vi "GxSingleCam.vi"() -> ()   [LabVIEW 2016]
uses:
  <vilib>/vision/Image Controls.llb/IMAQ Image.ctl
  GxLVLib/GxLVLib.lvlib
panel:
  in  "TriggerMode":string(combo)
  in  "Image Path":path
  in  "Image Src":T1
  out "IsColor":bool
  out "error out":errorcluster
  in  "DeviceHandle":u64
  out "IsExit":bool
  in  "ImageSaving":bool caption="保存图片"
  out "Acquisition Status":bool
  out "Open Status":bool
  in  "Exit":bool caption="安全退出"
  in  "TriggerSoftware":bool caption="发送软触发"
  in  "BalanceWhiteAuto":string(combo) caption="自动白平衡"
  in  "Gain":dbl caption="增益" format="%#_6f"
  in  "ExposureTime":dbl caption="曝光时间"
  in  "TriggerSource":string(combo) caption="触发源"
  in  "Acquisition Stop":bool caption="停止采集"
  in  "Acquisition Start":bool caption="开始采集"
  in  "Close Device":bool caption="关闭设备"
  in  "Open Device":bool caption="打开设备"
  out "Image":T1(plugin-control)
  # "TriggerMode"
  # "TriggerSource"
  # "TriggerSoftware"
  # "ExposureTime(us)"
  # "Gain(dB)"
  # "BalanceWhiteAuto"
  # "ImageSaving"
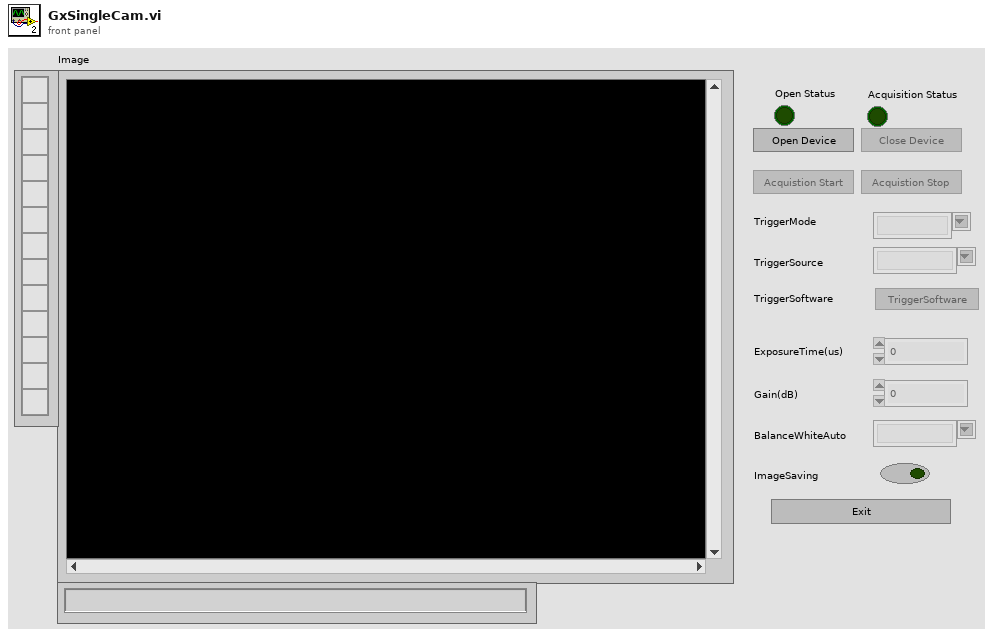
[diagram p1: front panel]
types:
  T1 = typedef "IMAQ Image.ctl" = refnum<image>
  T2 = typedef "Semaphore RefNum" = refnum<k1>
  T3 = cluster{"nFrameID":u64, "nTimestamp":u64, "nBufID":u64, "pImgBuf":u64, "nStatus":i32, "nWidth":i32, "nHeight":i32, "nPixelFormat":i32, "nImgSize":i32, "nOffsetX":i32, "nOffsetY":i32, "pUserParam":i32, cluster{"[0]":i32, "[1]":i32, "[2]":i32, "[3]":i32, "[4]":i32, "[5]":i32, "[6]":i32, "[7]":i32, "[8]":i32, "[9]":i32, "[10]":i32, "[11]":i32, "[12]":i32, "[13]":i32, "[14]":i32, "[15]":i32, "[16]":i32, "[17]":i32, "[18]":i32, "[19]":i32, "[20]":i32, "[21]":i32, "[22]":i32}}
  T4 = enum8{"Enabled", "Disabled", "Disabled and Grayed Out"}
  T5 = typedef "Image Type" = u32
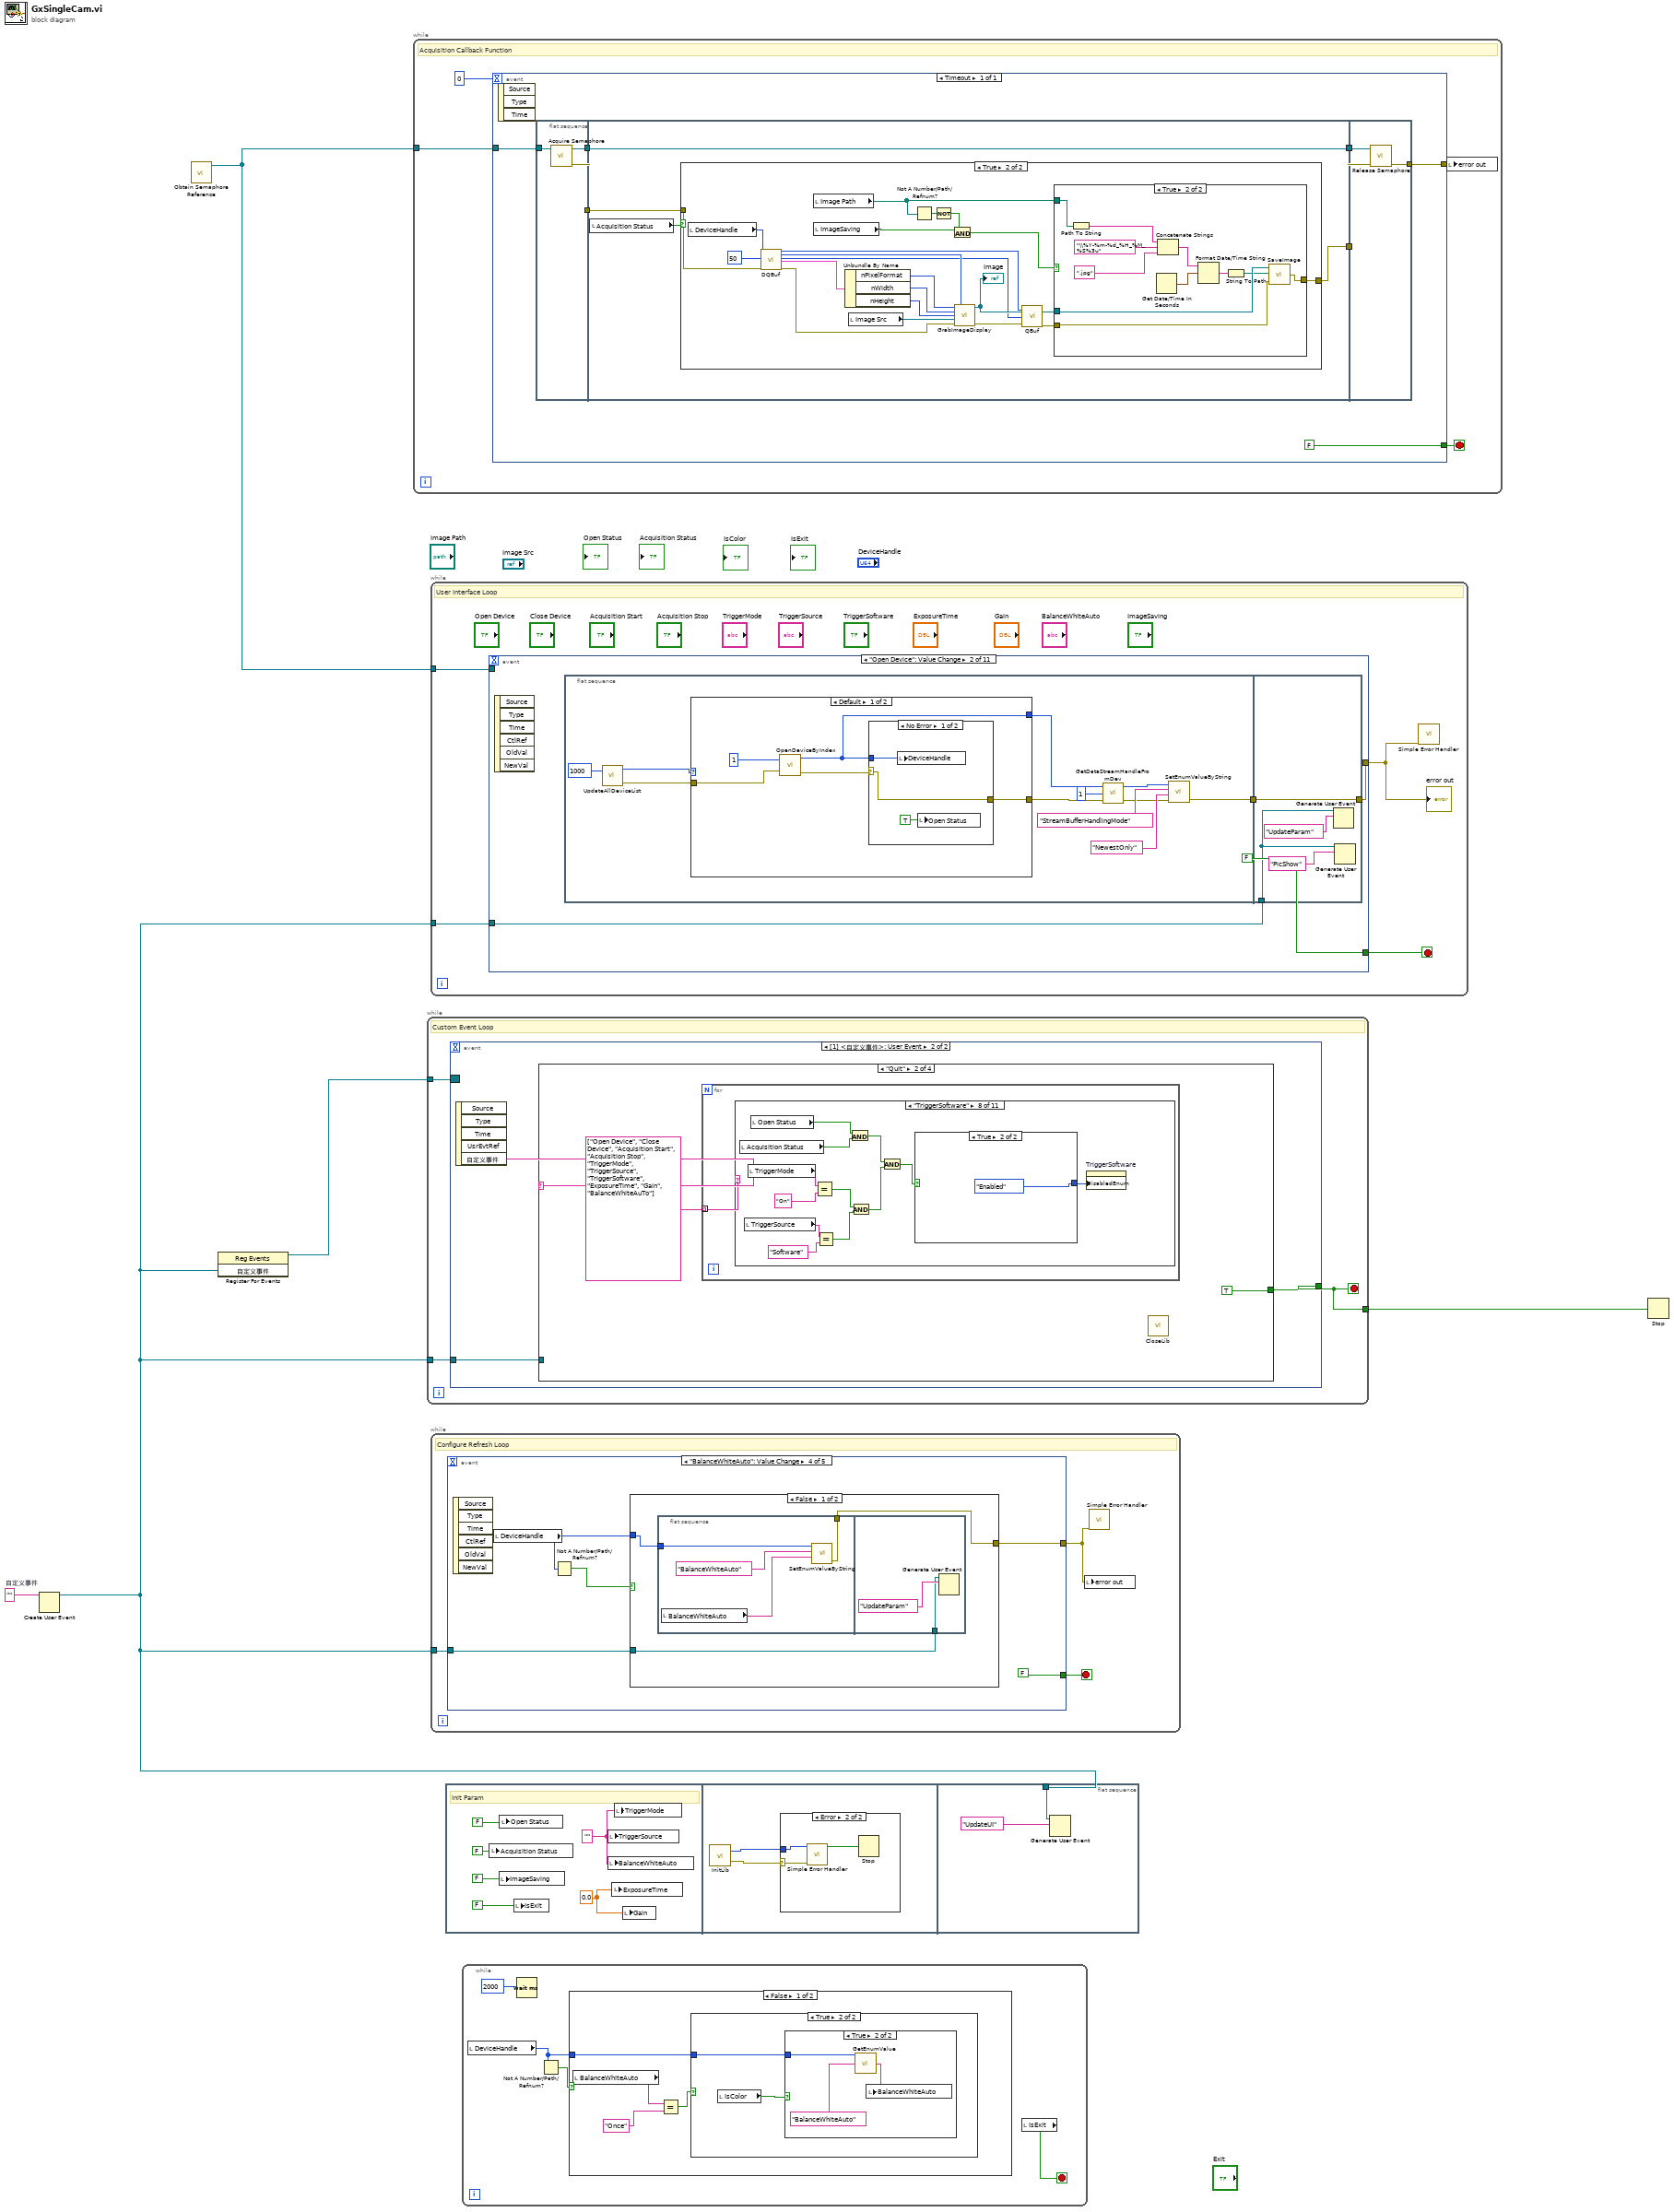
[diagram p0: block diagram]
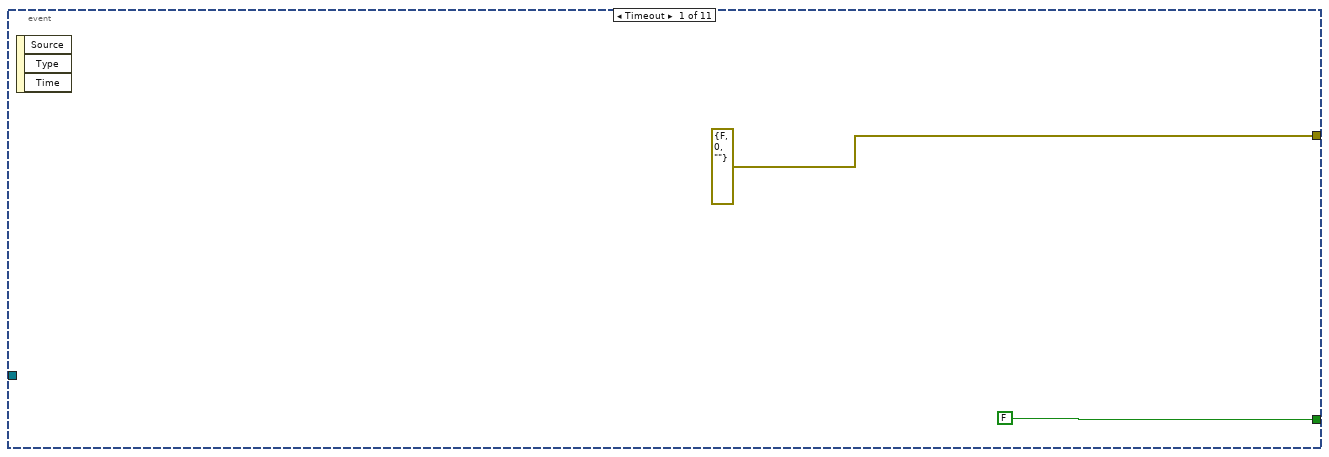
[diagram p4: hidden frame]
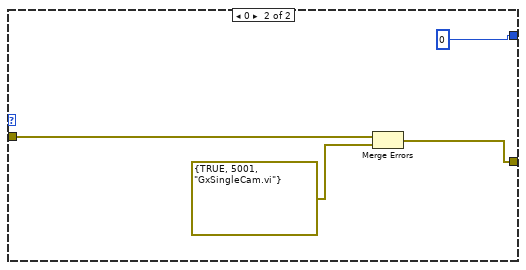
[diagram p6: hidden frame]
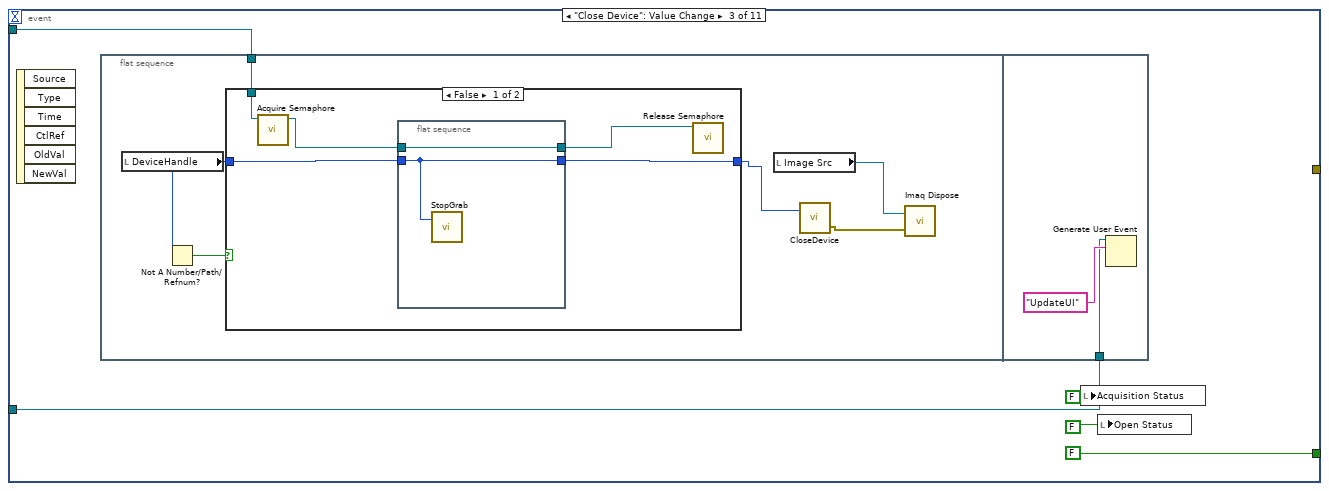
[diagram p7: hidden frame]
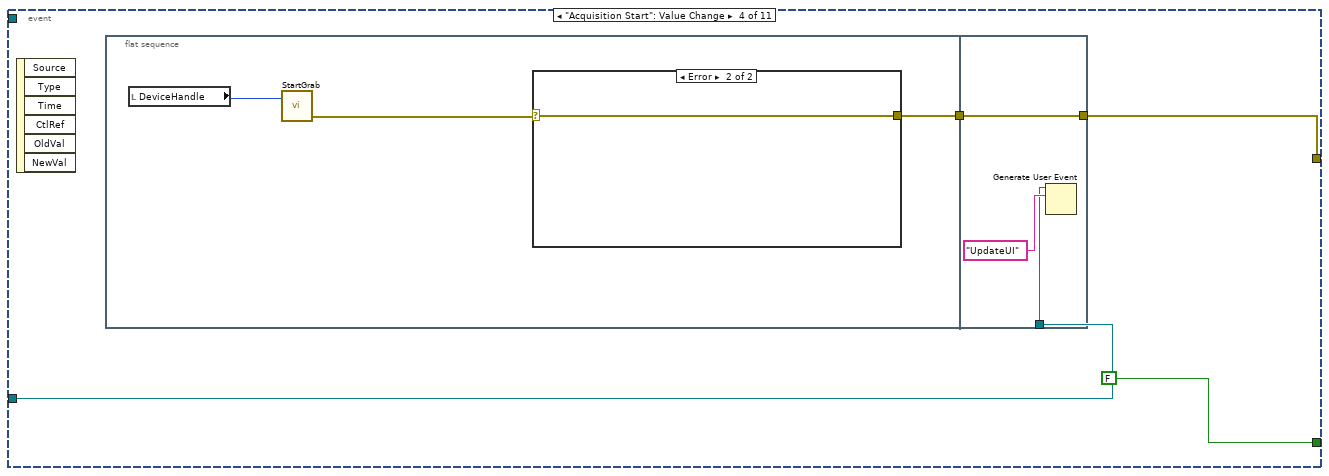
[diagram p9: hidden frame]
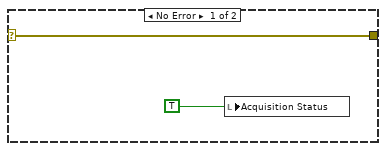
[diagram p10: hidden frame]
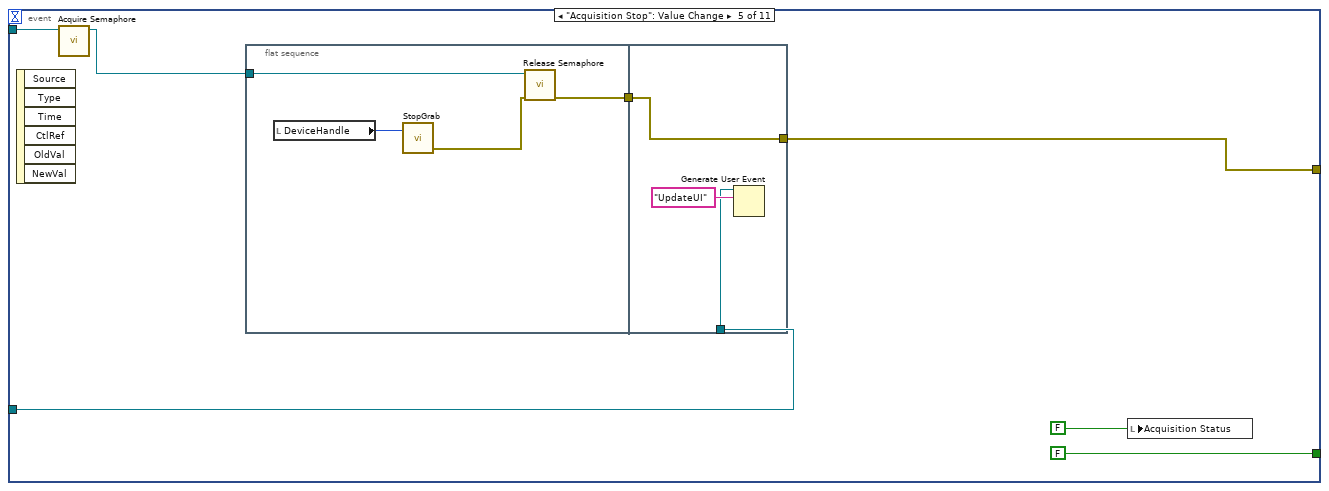
[diagram p11: hidden frame]
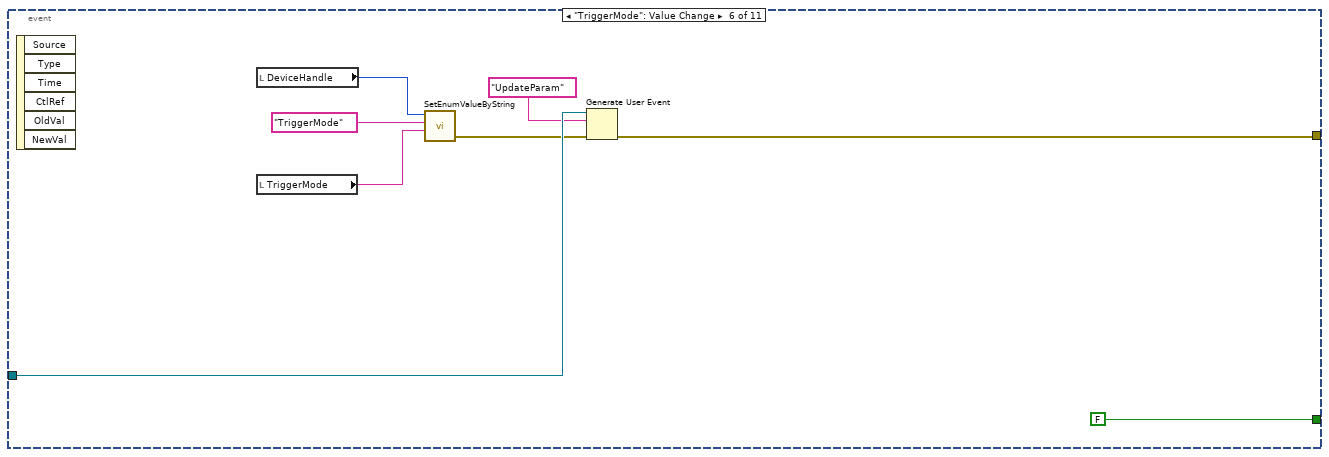
[diagram p12: hidden frame]
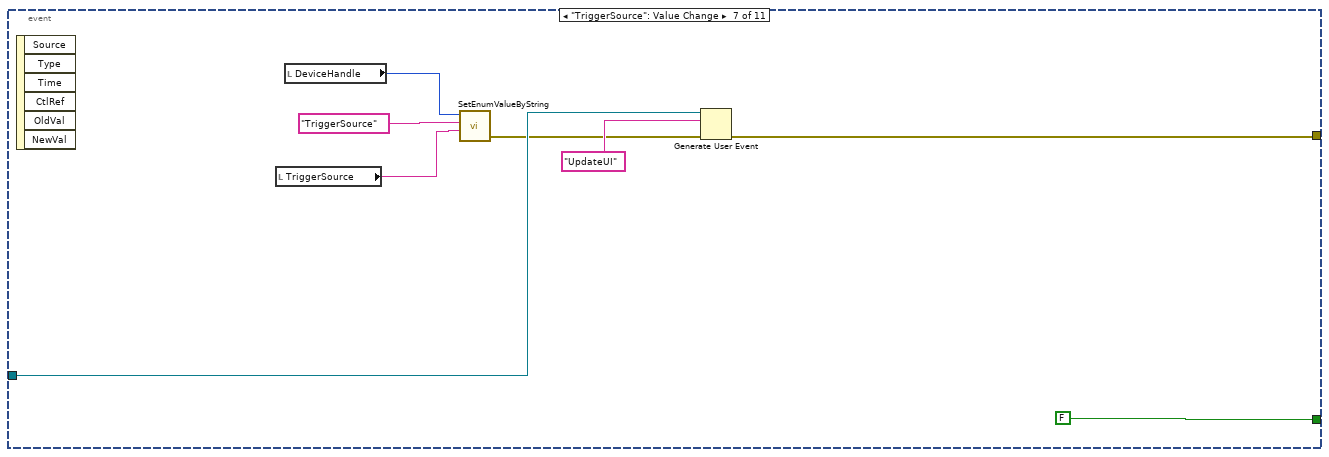
[diagram p13: hidden frame]
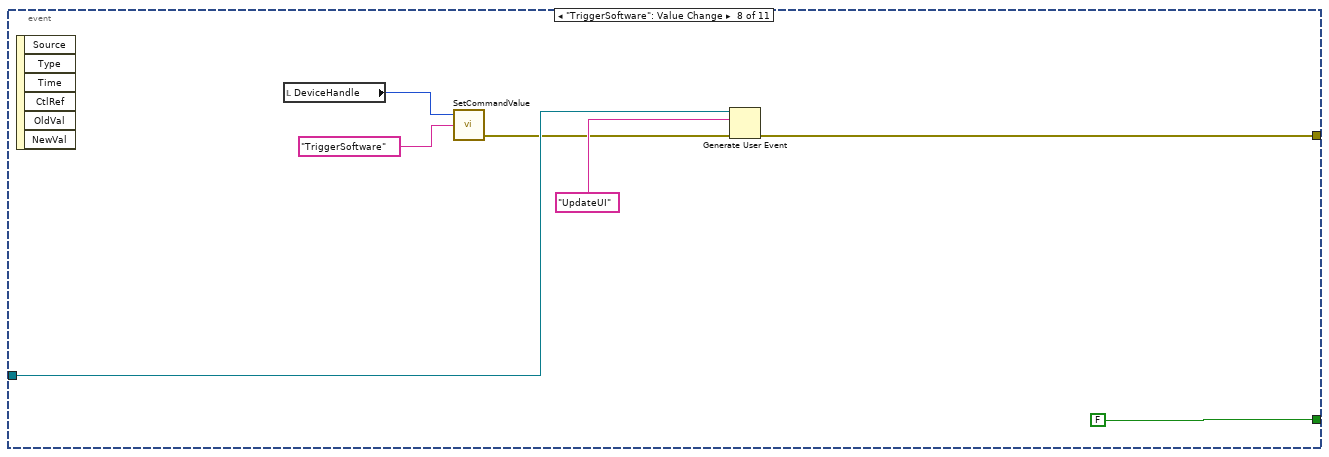
[diagram p14: hidden frame]
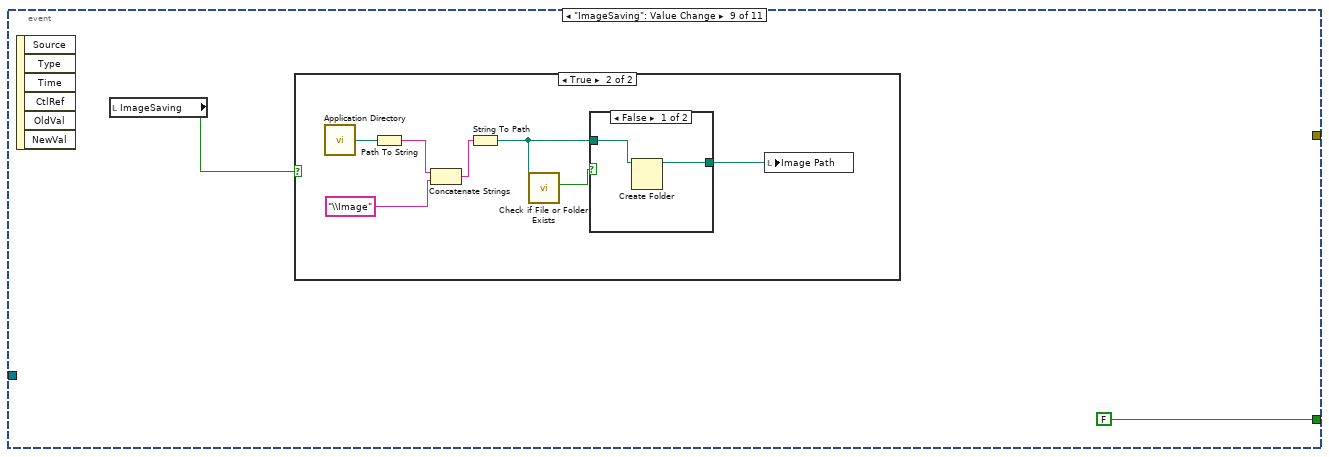
[diagram p15: hidden frame]
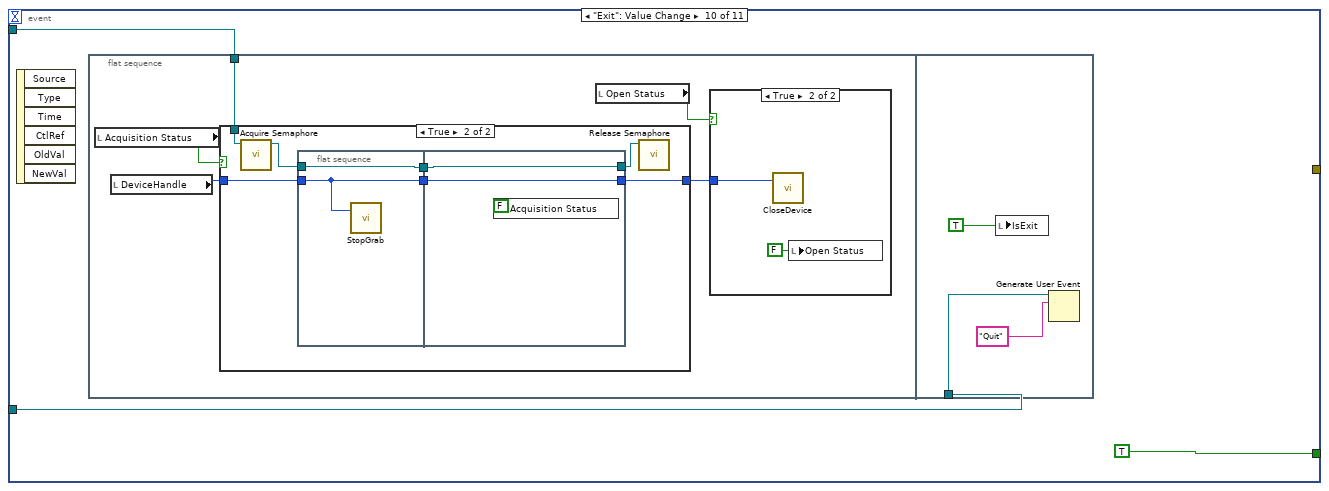
[diagram p18: hidden frame]
diagram:
  w5 = ""  # 自定义事件
  n1 = Create User Event(user event datatype=w5) -> (user event=w2:refnum<user-event>)  [unwired: 1 in, 1 out]
  n2 = call <vilib>:"Obtain Semaphore Reference.vi"() -> ("semaphore"=w1:T2)  [unwired: 5 in, 2 out]
  n3 = register-events(w2) -> (reference out=w4:refnum<event-registration>)  [unwired: 2 in, 1 out]
  n4 = while {
    tunnel: w1 -> [w6]
    stop <- w9 stop-if-true
    # "Acquisition Callback Function"
    n5 = event shown="[0] Timeout" {
      selector: _ -> [_]
      dyn-events: _ -> [_]
      timeout: 0 -> [_]
      tunnel: [FALSE] -> w9
      tunnel: [w15] -> w8
      tunnel: w6 -> [w14]
      event Timeout {
        n6 = event-data() -> ()  [unwired: 1 in, 3 out]
        n7 = flat-sequence {
          tunnel: w14 -> [w19]
          tunnel: [w18] -> w11
          tunnel: [w17] -> w10
          tunnel: [w23] -> w13
          tunnel: [w22] -> w12
          tunnel: w11 -> [w22]
          tunnel: w10 -> [w21]
          tunnel: [w58] -> w15
          tunnel: w13 -> [w59]
          tunnel: w12 -> [w60]
          frame #0 {
            n8 = call <vilib>:"Acquire Semaphore.vi"("semaphore"=w19) -> ("error out"=w17:errorcluster, "semaphore out"=w18:T2)  [unwired: 4 in, 1 out]
          }
          frame #1 {
            n9 = local read "Acquisition Status"() -> (w20:bool)
            n10 = case shown="True" w20 {
              tunnel: [w24 w40] -> w23
              tunnel: w21 -> [w24 w43]
              frame False {
              }
              frame True {
                n11 = local read "DeviceHandle"() -> (w45:u64)
                n12 = call "DQBuf.vi"("nInputHandle"=w45, "nTimeOut"=50, "error in (no error)"=w43) -> ("nOutputHandle"=w42:u64, "ImgBuf"=w32:u8[], "ppFrameBuffer"=w25:u64, "Dst"=w41:T3, "error out"=w28:errorcluster)  [unwired: 11 in, 1 out]
                n13 = local read "Image Path"() -> (w36:path)
                n14 = local read "ImageSaving"() -> (w35:bool)
                n15 = Unbundle By Name(w41) -> ("nPixelFormat"=w29:i32, "nWidth"=w31:i32, "nHeight"=w30:i32)
                n16 = local read "Image Src"() -> (w33:T1)
                n17 = Not A Number/Path/Refnum?(number/path/refnum=w36) -> (NaN/Path/Refnum?=w37:bool)
                n18 = Not(x=w37) -> (.not. x?=w38:bool)
                n19 = And(x=w35, y=w38) -> (x .and. y?=w34:bool)
                n20 = call "GrabImageDisplay.vi"("nPixelFormat"=w29, "pInputBuffer"=w32, "nWidth"=w31, "nHeight"=w30, "Image Src"=w33, "error in (no error)"=w28) -> ("Image out"=w27:T1, "error out"=w26:errorcluster)  [unwired: 8 in]
                "Image" <- w27
                n21 = call "QBuf.vi"("error in (no error)"=w26, "pBufferHandle"=w25, "nInputHandle"=w42) -> ("error out"=w39:errorcluster)  [unwired: 2 out]
                n22 = case shown="True" w34 {
                  tunnel: w36 -> [_ w53]
                  tunnel: w27 -> [_ w52]
                  tunnel: w39 -> [w46 w50]
                  tunnel: [w46 w49] -> w40
                  frame False {
                  }
                  frame True {
                    n23 = Path To String(path=w53) -> (string=w54:string)
                    n24 = Get Date/Time In Seconds() -> (seconds since 1Jan1904=w56:timestamp)
                    n25 = Concatenate Strings(w54, "\\%Y-%m-%d_%H_%M_%S%3u", ".jpg") -> (w55:string)
                    n26 = Format Date/Time String(time format string (%c)=w55, seconds (now)=w56) -> (date/time string=w57:string)  [unwired: 1 in]
                    n27 = String To Path(string=w57) -> (path=w51:path)
                    n28 = call "SaveImage.vi"("error in (no error)"=w50, "Path"=w51, "Image Src"=w52) -> ("error out"=w49:errorcluster)
                  }
                }
              }
            }
          }
          frame #2 {
            n29 = call <vilib>:"Release Semaphore.vi"("error in (no error)"=w59, "semaphore"=w60) -> ("error out"=w58:errorcluster)  [unwired: 4 in, 1 out]
          }
        }
      }
    }
    n30 = local write "error out"(w8) -> ()
  }
  n31 = while {
    tunnel: w4 -> [w63]
    tunnel: w2 -> [w62]
    tunnel: [w61] -> w3
    stop <- w61 stop-if-true
    # "Custom Event Loop"
    n32 = event shown="[1] <自定义事件>: User Event" {
      selector: w63 -> [_ _]
      dyn-events: _ -> [_ _]
      timeout: _ -> [_ _]
      tunnel: [FALSE w65] -> w61
      tunnel: w62 -> [_ w66]
      event Timeout {
        n33 = event-data() -> ()  [unwired: 1 in, 3 out]
      }
      event User Event {
        n34 = event-data() -> ("自定义事件"=w67:string)  [unwired: 1 in, 4 out]
        n35 = case shown="\"Quit\"" w67 {
          tunnel: w66 -> [_ _ w196 _]
          tunnel: [FALSE TRUE FALSE FALSE] -> w65
          frame "UpdateUI", Default {
            n36 = for {
              tunnel: string[] ["OpenDevice", "CloseDevice", "Acquisition Start", "Acquisition Stop", "TriggerMode", "TriggerSource", "TriggerSoftware", "ExposureTime", "Gain", "BalanceWhiteAuto"] -> [w70] mode=indexing
              n37 = case shown="\"BalanceWhiteAuto\"" w70 {
                frame Default {
                }
                frame "OpenDevice" {
                  n38 = local read "Open Status"() -> (w72:bool)
                  n39 = case shown="True" w72 {
                    tunnel: [T4."Enabled" ("禁用") T4."Disabled and Grayed Out" ("禁用")] -> w71
                    frame False {
                    }
                    frame True {
                    }
                  }
                  n40 = property on="Open Device" class="Bool"("DisabledEnum"=w71) -> ()  [unwired: 2 in, 2 out]
                }
                frame "CloseDevice" {
                  n41 = local read "Open Status"() -> (w76:bool)
                  n42 = case shown="True" w76 {
                    tunnel: [T4."Disabled and Grayed Out" ("禁用") T4."Enabled" ("禁用")] -> w75
                    frame False {
                    }
                    frame True {
                    }
                  }
                  n43 = property on="Close Device" class="Bool"("DisabledEnum"=w75) -> ()  [unwired: 2 in, 2 out]
                }
                frame "Acquisition Start" {
                  n44 = local read "Acquisition Status"() -> (w83:bool)
                  n45 = local read "Open Status"() -> (w82:bool)
                  n46 = Not(x=w83) -> (.not. x?=w81:bool)
                  n47 = And(x=w82, y=w81) -> (x .and. y?=w80:bool)
                  n48 = case shown="False" w80 {
                    tunnel: [T4."Disabled and Grayed Out" ("禁用") T4."Enabled" ("禁用")] -> w79
                    frame False {
                    }
                    frame True {
                    }
                  }
                  n49 = property on="Acquisition Start" class="Bool"("DisabledEnum"=w79) -> ()  [unwired: 2 in, 2 out]
                }
                frame "Acquisition Stop" {
                  n50 = local read "Acquisition Status"() -> (w87:bool)
                  n51 = case shown="False" w87 {
                    tunnel: [T4."Disabled and Grayed Out" ("禁用") T4."Enabled" ("禁用")] -> w86
                    frame False {
                    }
                    frame True {
                    }
                  }
                  n52 = property on="Acquisition Stop" class="Bool"("DisabledEnum"=w86) -> ()  [unwired: 2 in, 2 out]
                }
                frame "TriggerMode" {
                  n53 = local read "Open Status"() -> (w91:bool)
                  n54 = case shown="True" w91 {
                    tunnel: [T4."Disabled and Grayed Out" ("禁用") T4."Enabled" ("禁用")] -> w90
                    frame False {
                    }
                    frame True {
                    }
                  }
                  n55 = property on="TriggerMode" class="CmbBox"("DisabledEnum"=w90) -> ()  [unwired: 2 in, 2 out]
                }
                frame "TriggerSource" {
                  n56 = local read "TriggerMode"() -> (w94:string)
                  n57 = local read "Open Status"() -> (w98:bool)
                  n58 = Equal?(x=w94, y="On") -> (x = y?=w97:bool)
                  n59 = And(x=w98, y=w97) -> (x .and. y?=w96:bool)
                  n60 = case shown="True" w96 {
                    tunnel: [T4."Disabled and Grayed Out" ("禁用") T4."Enabled" ("禁用")] -> w95
                    frame False {
                    }
                    frame True {
                    }
                  }
                  n61 = property on="TriggerSource" class="CmbBox"("DisabledEnum"=w95) -> ()  [unwired: 2 in, 2 out]
                }
                frame "TriggerSoftware" {
                  n62 = local read "Acquisition Status"() -> (w103:bool)
                  n63 = local read "TriggerSource"() -> (w111:string)
                  n64 = local read "TriggerMode"() -> (w113:string)
                  n65 = local read "Open Status"() -> (w104:bool)
                  n66 = Equal?(x=w113, y="On") -> (x = y?=w109:bool)
                  n67 = Equal?(x=w111, y="Software") -> (x = y?=w108:bool)
                  n68 = And(x=w104, y=w103) -> (x .and. y?=w102:bool)
                  n69 = And(x=w109, y=w108) -> (x .and. y?=w107:bool)
                  n70 = And(x=w102, y=w107) -> (x .and. y?=w106:bool)
                  n71 = case shown="True" w106 {
                    tunnel: [T4."Disabled and Grayed Out" ("禁用") T4."Enabled" ("禁用")] -> w105
                    frame False {
                    }
                    frame True {
                    }
                  }
                  n72 = property on="TriggerSoftware" class="Bool"("DisabledEnum"=w105) -> ()  [unwired: 2 in, 2 out]
                }
                frame "ExposureTime" {
                  n73 = local read "Open Status"() -> (w117:bool)
                  n74 = case shown="False" w117 {
                    tunnel: [T4."Disabled and Grayed Out" ("禁用") T4."Enabled" ("禁用")] -> w116
                    frame False {
                    }
                    frame True {
                    }
                  }
                  n75 = property on="ExposureTime" class="DigNum (strict)"("DisabledEnum"=w116) -> ()  [unwired: 2 in, 2 out]
                }
                frame "Gain" {
                  n76 = local read "Open Status"() -> (w121:bool)
                  n77 = case shown="True" w121 {
                    tunnel: [T4."Disabled and Grayed Out" ("禁用") T4."Enabled" ("禁用")] -> w120
                    frame False {
                    }
                    frame True {
                    }
                  }
                  n78 = property on="Gain" class="DigNum (strict)"("DisabledEnum"=w120) -> ()  [unwired: 2 in, 2 out]
                }
                frame "BalanceWhiteAuto" {
                  n79 = local read "Open Status"() -> (w126:bool)
                  n80 = local read "IsColor"() -> (w127:bool)
                  n81 = And(x=w126, y=w127) -> (x .and. y?=w125:bool)
                  n82 = case shown="True" w125 {
                    tunnel: [T4."Disabled and Grayed Out" ("禁用") T4."Enabled" ("禁用")] -> w124
                    frame False {
                    }
                    frame True {
                    }
                  }
                  n83 = property on="BalanceWhiteAuto" class="CmbBox"("DisabledEnum"=w124) -> ()  [unwired: 2 in, 2 out]
                }
              }
            }
          }
          frame "Quit" {
            n84 = for {
              tunnel: string[] ["Open Device", "Close Device", "Acquisition Start", "Acquisition Stop", "TriggerMode", "TriggerSource", "TriggerSoftware", "ExposureTime", "Gain", "BalanceWhiteAuTo"] -> [w132] mode=indexing
              n85 = case shown="\"TriggerSoftware\"" w132 {
                frame Default {
                }
                frame "Open Device" {
                  n86 = local read "Open Status"() -> (w134:bool)
                  n87 = case shown="True" w134 {
                    tunnel: [T4."Enabled" ("禁用") T4."Disabled and Grayed Out" ("禁用")] -> w133
                    frame False {
                    }
                    frame True {
                    }
                  }
                  n88 = property on="Open Device" class="Bool"("DisabledEnum"=w133) -> ()  [unwired: 2 in, 2 out]
                }
                frame "Close Device" {
                  n89 = local read "Open Status"() -> (w138:bool)
                  n90 = case shown="False" w138 {
                    tunnel: [T4."Disabled and Grayed Out" ("禁用") T4."Enabled" ("禁用")] -> w137
                    frame False {
                    }
                    frame True {
                    }
                  }
                  n91 = property on="Close Device" class="Bool"("DisabledEnum"=w137) -> ()  [unwired: 2 in, 2 out]
                }
                frame "Acquisition Start" {
                  n92 = local read "Acquisition Status"() -> (w145:bool)
                  n93 = local read "Open Status"() -> (w144:bool)
                  n94 = Not(x=w145) -> (.not. x?=w143:bool)
                  n95 = And(x=w144, y=w143) -> (x .and. y?=w142:bool)
                  n96 = case shown="False" w142 {
                    tunnel: [T4."Disabled and Grayed Out" ("禁用") T4."Enabled" ("禁用")] -> w141
                    frame False {
                    }
                    frame True {
                    }
                  }
                  n97 = property on="Acquisition Start" class="Bool"("DisabledEnum"=w141) -> ()  [unwired: 2 in, 2 out]
                }
                frame "Acquisition Stop" {
                  n98 = local read "Acquisition Status"() -> (w149:bool)
                  n99 = case shown="True" w149 {
                    tunnel: [T4."Disabled and Grayed Out" ("禁用") T4."Enabled" ("禁用")] -> w148
                    frame False {
                    }
                    frame True {
                    }
                  }
                  n100 = property on="Acquisition Stop" class="Bool"("DisabledEnum"=w148) -> ()  [unwired: 2 in, 2 out]
                }
                frame "TriggerMode" {
                  n101 = local read "Open Status"() -> (w153:bool)
                  n102 = case shown="True" w153 {
                    tunnel: [T4."Disabled and Grayed Out" ("禁用") T4."Enabled" ("禁用")] -> w152
                    frame False {
                    }
                    frame True {
                    }
                  }
                  n103 = property on="TriggerMode" class="CmbBox"("DisabledEnum"=w152) -> ()  [unwired: 2 in, 2 out]
                }
                frame "TriggerSource" {
                  n104 = local read "TriggerMode"() -> (w156:string)
                  n105 = local read "Open Status"() -> (w160:bool)
                  n106 = Equal?(x=w156, y="On") -> (x = y?=w159:bool)
                  n107 = And(x=w160, y=w159) -> (x .and. y?=w158:bool)
                  n108 = case shown="False" w158 {
                    tunnel: [T4."Disabled and Grayed Out" ("禁用") T4."Enabled" ("禁用")] -> w157
                    frame False {
                    }
                    frame True {
                    }
                  }
                  n109 = property on="TriggerSource" class="CmbBox"("DisabledEnum"=w157) -> ()  [unwired: 2 in, 2 out]
                }
                frame "TriggerSoftware" {
                  n110 = local read "Acquisition Status"() -> (w165:bool)
                  n111 = local read "TriggerSource"() -> (w173:string)
                  n112 = local read "TriggerMode"() -> (w175:string)
                  n113 = local read "Open Status"() -> (w166:bool)
                  n114 = Equal?(x=w175, y="On") -> (x = y?=w171:bool)
                  n115 = Equal?(x=w173, y="Software") -> (x = y?=w170:bool)
                  n116 = And(x=w166, y=w165) -> (x .and. y?=w164:bool)
                  n117 = And(x=w171, y=w170) -> (x .and. y?=w169:bool)
                  n118 = And(x=w164, y=w169) -> (x .and. y?=w168:bool)
                  n119 = case shown="True" w168 {
                    tunnel: [T4."Disabled and Grayed Out" ("禁用") T4."Enabled" ("禁用")] -> w167
                    frame False {
                    }
                    frame True {
                    }
                  }
                  n120 = property on="TriggerSoftware" class="Bool"("DisabledEnum"=w167) -> ()  [unwired: 2 in, 2 out]
                }
                frame "ExposureTime" {
                  n121 = local read "Open Status"() -> (w179:bool)
                  n122 = case shown="False" w179 {
                    tunnel: [T4."Disabled and Grayed Out" ("禁用") T4."Enabled" ("禁用")] -> w178
                    frame False {
                    }
                    frame True {
                    }
                  }
                  n123 = property on="ExposureTime" class="DigNum (strict)"("DisabledEnum"=w178) -> ()  [unwired: 2 in, 2 out]
                }
                frame "Gain" {
                  n124 = local read "Open Status"() -> (w183:bool)
                  n125 = case shown="True" w183 {
                    tunnel: [T4."Disabled and Grayed Out" ("禁用") T4."Enabled" ("禁用")] -> w182
                    frame False {
                    }
                    frame True {
                    }
                  }
                  n126 = property on="Gain" class="DigNum (strict)"("DisabledEnum"=w182) -> ()  [unwired: 2 in, 2 out]
                }
                frame "BalanceWhiteAuto" {
                  n127 = local read "Open Status"() -> (w188:bool)
                  n128 = local read "IsColor"() -> (w189:bool)
                  n129 = And(x=w188, y=w189) -> (x .and. y?=w187:bool)
                  n130 = case shown="True" w187 {
                    tunnel: [T4."Disabled and Grayed Out" ("禁用") T4."Enabled" ("禁用")] -> w186
                    frame False {
                    }
                    frame True {
                    }
                  }
                  n131 = property on="BalanceWhiteAuto" class="CmbBox"("DisabledEnum"=w186) -> ()  [unwired: 2 in, 2 out]
                }
              }
            }
            n132 = call "CloseLib.vi"() -> ()  [unwired: 1 in, 2 out]
          }
          frame "UpdateParam" {
            n133 = local read "DeviceHandle"() -> (w198:u64)
            n134 = local read "Open Status"() -> (w202:bool)
            n135 = Not A Number/Path/Refnum?(number/path/refnum=w198) -> (NaN/Path/Refnum?=w199:bool)
            n136 = Not(x=w199) -> (.not. x?=w201:bool)
            n137 = And(x=w201, y=w202) -> (x .and. y?=w200:bool)
            n138 = case shown="True" w200 {
              tunnel: [errorcluster {FALSE, 0, ""} w204] -> w195
              tunnel: string[] ["TriggerMode", "TriggerSource", "ExposureTime", "Gain", "BalanceWhiteAuto"] -> [_ w207]
              tunnel: w198 -> [_ w206]
              frame False {
              }
              frame True {
                n139 = for {
                  tunnel: w207 -> [w210] mode=indexing
                  tunnel: w206 -> [w209]
                  tunnel: [w208] -> w205 mode=indexing
                  n140 = case shown="\"BalanceWhiteAuto\"" w210 {
                    selector: w210 -> [w213 w218 w221 w225 w230]
                    tunnel: w209 -> [w211 w215 w220 w224 w229]
                    tunnel: [w214 w217 w222 w226 w232] -> w208
                    frame "TriggerMode", Default {
                      n141 = call "GetEnumValue.vi"("nInputHandle"=w211, "strName"=w213) -> ("strCurName"=w212:string, "error out"=w214:errorcluster)  [unwired: 9 in, 3 out]
                      n142 = local write "TriggerMode"(w212) -> ()
                    }
                    frame "TriggerSource" {
                      n143 = call "GetEnumValue.vi"("nInputHandle"=w215, "strName"=w218) -> ("strCurName"=w216:string, "error out"=w217:errorcluster)  [unwired: 9 in, 3 out]
                      n144 = local write "TriggerSource"(w216) -> ()
                    }
                    frame "ExposureTime" {
                      n145 = call "GetFloatValue.vi"("nInputHandle"=w220, "strName"=w221) -> ("dCurValue"=w219:dbl, "error out"=w222:errorcluster)  [unwired: 9 in, 3 out]
                      n146 = local write "ExposureTime"(w219) -> ()
                    }
                    frame "Gain" {
                      n147 = call "GetFloatValue.vi"("nInputHandle"=w224, "strName"=w225) -> ("dCurValue"=w223:dbl, "error out"=w226:errorcluster)  [unwired: 9 in, 3 out]
                      n148 = local write "Gain"(w223) -> ()
                    }
                    frame "BalanceWhiteAuto" {
                      n149 = call "IsImplemented.vi"("strName"=w230, "Read Data"=FALSE, "nInputHandle"=w229) -> ("error out"=w231:errorcluster, "Result"=w227:bool)  [unwired: 1 in, 2 out]
                      n150 = case shown="True" w227 {
                        tunnel: [w233 w238] -> w232
                        tunnel: w231 -> [w233 w236]
                        tunnel: w229 -> [_ w234]
                        tunnel: w230 -> [_ w235]
                        frame False {
                        }
                        frame True {
                          n151 = call "GetEnumValue.vi"("nInputHandle"=w234, "strName"=w235, "error in (no error)"=w236) -> ("strCurName"=w237:string, "error out"=w238:errorcluster)  [unwired: 8 in, 3 out]
                          n152 = local write "BalanceWhiteAuto"(w237) -> ()
                        }
                      }
                      n153 = local write "IsColor"(w227) -> ()
                    }
                  }
                }
                n154 = Merge Errors(w205) -> (w204:errorcluster)
              }
            }
            n155 = Generate User Event(user event=w196, event data cluster="UpdateUI", error in=w195) -> (error out=w194:errorcluster)  [unwired: 1 in, 1 out]
            n156 = local write "error out"(w194) -> ()
            n157 = call <vilib>:"Simple Error Handler.vi"("error in (no error)"=w194) -> ()  [unwired: 4 in, 5 out]
          }
          frame "PicShow" {
            n158 = local read "DeviceHandle"() -> (w241:u64)
            n159 = local read "Open Status"() -> (w245:bool)
            n160 = Not A Number/Path/Refnum?(number/path/refnum=w241) -> (NaN/Path/Refnum?=w242:bool)
            n161 = Not(x=w242) -> (.not. x?=w244:bool)
            n162 = And(x=w244, y=w245) -> (x .and. y?=w243:bool)
            n163 = case shown="True" w243 {
              tunnel: [errorcluster {FALSE, 0, ""} errorcluster {FALSE, 0, ""}] -> w239
              tunnel: w241 -> [_ w250]
              frame False {
              }
              frame True {
                n164 = call "IsImplemented.vi"("strName"="PixelColorFilter", "Read Data"=TRUE, "nInputHandle"=w250) -> ("Result"=w247:bool)  [unwired: 1 in, 3 out]
                n165 = case shown="True" w247 {
                  tunnel: w250 -> [_ w258]
                  tunnel: [w255 w259] -> w252
                  frame False {
                    w255 = T5 0 items=["Grayscale (U8)", "Grayscale (I16)", "Grayscale (SGL)", "Complex (CSG)", "RGB (U32)", "HSL (U32)", "RGB (U64)", "Grayscale (U16)"] ("Image Type")
                  }
                  frame True {
                    n166 = call "GetEnumValue.vi"("nInputHandle"=w258, "strName"="PixelColorFilter") -> ("strCurName"=w256:string)  [unwired: 9 in, 4 out]
                    n167 = Equal?(x=w256, y="None") -> (x = y?=w260:bool)
                    n168 = case shown="True" w260 {
                      tunnel: [w262 w263] -> w259
                      frame False {
                        w262 = T5 4 items=["Grayscale (U8)", "Grayscale (I16)", "Grayscale (SGL)", "Complex (CSG)", "RGB (U32)", "HSL (U32)", "RGB (U64)", "Grayscale (U16)"] ("Image Type")
                      }
                      frame True {
                        w263 = T5 0 items=["Grayscale (U8)", "Grayscale (I16)", "Grayscale (SGL)", "Complex (CSG)", "RGB (U32)", "HSL (U32)", "RGB (U64)", "Grayscale (U16)"] ("Image Type")
                      }
                    }
                  }
                }
                n169 = call "IMAQ Create"("Image Name"="", "Image Type"=w252) -> ("New Image"=w253:T1)  [unwired: 3 in, 1 out]
                n170 = local write "Image Src"(w253) -> ()
              }
            }
            n171 = local write "error out"(w239) -> ()
            n172 = call <vilib>:"Simple Error Handler.vi"("error in (no error)"=w239) -> ()  [unwired: 4 in, 5 out]
          }
        }
      }
    }
  }
  n173 = while {
    tunnel: w2 -> [w267]
    tunnel: w1 -> [w265]
    stop <- w266 stop-if-true
    # "User Interface Loop"
    n174 = event shown="[1] \"Open Device\": Value Change" {
      selector: _ -> [_ _ _ _ _ _ _ _ _ _ _]
      dyn-events: _ -> [_ _ _ _ _ _ _ _ _ _ _]
      timeout: _ -> [_ _ _ _ _ _ _ _ _ _ _]
      tunnel: [errorcluster {FALSE, 0, ""} w272 _ w325 w337 w355 w363 w369 _ _ _] -> w264
      tunnel: [FALSE FALSE FALSE FALSE FALSE FALSE FALSE FALSE FALSE TRUE TRUE] -> w266
      tunnel: w267 -> [_ w271 w303 w323 w338 w356 w364 w371 _ w386 w412]
      tunnel: w265 -> [_ _ w302 _ w341 _ _ _ _ w385 w411]
      event Timeout {
        n175 = event-data() -> ()  [unwired: 1 in, 3 out]
      }
      event "Open Device": Value Change {
        n176 = event-data() -> ()  [unwired: 1 in, 6 out]
        n177 = flat-sequence {
          tunnel: [w275] -> w270
          tunnel: [w301] -> w272
          tunnel: w271 -> [w298]
          tunnel: w270 -> [w301]
          frame #0 {
            n178 = call "UpdateAllDeviceList.vi"("nTimeOut"=1000) -> ("punNumDevices"=w282:i32, "error out"=w283:errorcluster)  [unwired: 1 in, 1 out]
            n179 = case shown="Default" w282 {
              tunnel: [w289 w296] -> w276
              tunnel: w283 -> [w288 w297]
              tunnel: [w285 0] -> w274
              frame Default {
                n180 = call "OpenDeviceByIndex.vi"("nDeviceIndex"=1 ("Index"), "error in (no error)"=w288) -> ("phDevice"=w285:u64, "error out"=w287:errorcluster)  [unwired: 1 out]
                n181 = case shown="No Error" w287 {
                  selector: w287 -> [w290 w293]
                  tunnel: w285 -> [w291 _]
                  tunnel: [w290 w293] -> w289
                  frame No Error {
                    n182 = local write "DeviceHandle"(w291) -> ()
                    n183 = local write "Open Status"(TRUE) -> ()
                  }
                  frame Error {
                  }
                }
              }
              frame 0 {
                n184 = Merge Errors(w297, errorcluster {TRUE, 5001, "GxSingleCam.vi"}) -> (w296:errorcluster)
              }
            }
            n185 = call "GetDataStreamHandleFromDev.vi"("error in (no error)"=w276, "DSIndex"=u32 1, "nInputHandle"=w274) -> ("error out"=w277:errorcluster, "phDS"=w280:u64)  [unwired: 1 out]
            n186 = call "SetEnumValueByString.vi"("error in (no error)"=w277, "strValue"="NewestOnly", "strName"="StreamBufferHandlingMode", "nInputHandle"=w280) -> ("error out"=w275:errorcluster)  [unwired: 2 out]
          }
          frame #1 {
            n187 = Generate User Event(user event=w298, event data cluster="UpdateParam") -> ()  [unwired: 2 in, 2 out]
            n188 = Generate User Event(user event=w298, event data cluster="PicShow") -> ()  [unwired: 2 in, 2 out]
          }
        }
      }
      event "Close Device": Value Change {
        n189 = event-data() -> ()  [unwired: 1 in, 6 out]
        n190 = flat-sequence {
          tunnel: w302 -> [w310]
          tunnel: w303 -> [w321]
          frame #0 {
            n191 = local read "DeviceHandle"() -> (w309:u64)
            n192 = Not A Number/Path/Refnum?(number/path/refnum=w309) -> (NaN/Path/Refnum?=w311:bool)
            n193 = case shown="False" w311 {
              tunnel: w309 -> [w317 w320]
              tunnel: [w316 w320] -> w308
              tunnel: w310 -> [w315 _]
              frame False {
                n194 = call <vilib>:"Acquire Semaphore.vi"("semaphore"=w315) -> ("semaphore out"=w314:T2)  [unwired: 4 in, 2 out]
                n195 = flat-sequence {
                  tunnel: w317 -> [w318]
                  tunnel: w314 -> [w319]
                  tunnel: [w318] -> w316
                  tunnel: [w319] -> w313
                  frame #0 {
                    n196 = call "StopGrab.vi"("InputHandle"=w318) -> ()  [unwired: 1 in, 3 out]
                  }
                }
                n197 = call <vilib>:"Release Semaphore.vi"("semaphore"=w313) -> ()  [unwired: 5 in, 2 out]
              }
              frame True {
              }
            }
            n198 = local read "Image Src"() -> (w312:T1)
            n199 = call "CloseDevice.vi"("nInputHandle"=w308) -> ("error out"=w307:errorcluster)  [unwired: 1 in, 1 out]
            n200 = call "Imaq Dispose"("Image"=w312, "error in (no error)"=w307) -> ()  [unwired: 1 in, 4 out]
          }
          frame #1 {
            n201 = Generate User Event(user event=w321, event data cluster="UpdateUI") -> ()  [unwired: 2 in, 2 out]
          }
        }
        n202 = local write "Acquisition Status"(FALSE) -> ()
        n203 = local write "Open Status"(FALSE) -> ()
      }
      event "Acquisition Start": Value Change {
        n204 = event-data() -> ()  [unwired: 1 in, 6 out]
        n205 = flat-sequence {
          tunnel: [w328] -> w324
          tunnel: [w335] -> w325
          tunnel: w324 -> [w335]
          tunnel: w323 -> [w333]
          frame #0 {
            n206 = local read "DeviceHandle"() -> (w329:u64)
            n207 = call "StartGrab.vi"("nInputHandle"=w329) -> ("error out"=w327:errorcluster)  [unwired: 1 in, 2 out]
            n208 = case shown="Error" w327 {
              selector: w327 -> [w331 w332]
              tunnel: [w331 w332] -> w328
              frame No Error {
                n209 = local write "Acquisition Status"(TRUE) -> ()
              }
              frame Error {
              }
            }
          }
          frame #1 {
            n210 = Generate User Event(user event=w333, event data cluster="UpdateUI") -> ()  [unwired: 2 in, 2 out]
          }
        }
      }
      event "Acquisition Stop": Value Change {
        n211 = event-data() -> ()  [unwired: 1 in, 6 out]
        n212 = call <vilib>:"Acquire Semaphore.vi"("semaphore"=w341) -> ("semaphore out"=w339:T2)  [unwired: 4 in, 2 out]
        n213 = flat-sequence {
          tunnel: w339 -> [w345]
          tunnel: [w344] -> w336
          tunnel: [w347] -> w337
          tunnel: w338 -> [w348]
          tunnel: w336 -> [w347]
          frame #0 {
            n214 = local read "DeviceHandle"() -> (w346:u64)
            n215 = call "StopGrab.vi"("InputHandle"=w346) -> ("error out"=w343:errorcluster)  [unwired: 1 in, 2 out]
            n216 = call <vilib>:"Release Semaphore.vi"("error in (no error)"=w343, "semaphore"=w345) -> ("error out"=w344:errorcluster)  [unwired: 4 in, 1 out]
          }
          frame #1 {
            n217 = Generate User Event(user event=w348, event data cluster="UpdateUI") -> ()  [unwired: 2 in, 2 out]
          }
        }
        n218 = local write "Acquisition Status"(FALSE) -> ()
      }
      event "TriggerMode": Value Change {
        n219 = event-data() -> ()  [unwired: 1 in, 6 out]
        n220 = local read "DeviceHandle"() -> (w351:u64)
        n221 = local read "TriggerMode"() -> (w353:string)
        n222 = call "SetEnumValueByString.vi"("strValue"=w353, "strName"="TriggerMode", "nInputHandle"=w351) -> ("error out"=w350:errorcluster)  [unwired: 1 in, 2 out]
        n223 = Generate User Event(user event=w356, event data cluster="UpdateParam", error in=w350) -> (error out=w355:errorcluster)  [unwired: 1 in, 1 out]
      }
      event "TriggerSource": Value Change {
        n224 = event-data() -> ()  [unwired: 1 in, 6 out]
        n225 = local read "TriggerSource"() -> (w359:string)
        n226 = local read "DeviceHandle"() -> (w361:u64)
        n227 = call "SetEnumValueByString.vi"("strValue"=w359, "strName"="TriggerSource", "nInputHandle"=w361) -> ("error out"=w358:errorcluster)  [unwired: 1 in, 2 out]
        n228 = Generate User Event(user event=w364, event data cluster="UpdateUI", error in=w358) -> (error out=w363:errorcluster)  [unwired: 1 in, 1 out]
      }
      event "TriggerSoftware": Value Change {
        n229 = event-data() -> ()  [unwired: 1 in, 6 out]
        n230 = local read "DeviceHandle"() -> (w367:u64)
        n231 = call "SetCommandValue.vi"("strName"="TriggerSoftware", "nInputHandle"=w367) -> ("error out"=w366:errorcluster)  [unwired: 1 in, 2 out]
        n232 = Generate User Event(user event=w371, event data cluster="UpdateUI", error in=w366) -> (error out=w369:errorcluster)  [unwired: 1 in, 1 out]
      }
      event "ImageSaving": Value Change {
        n233 = event-data() -> ()  [unwired: 1 in, 6 out]
        n234 = local read "ImageSaving"() -> (w374:bool)
        n235 = case shown="True" w374 {
          frame False {
          }
          frame True {
            n236 = call <vilib>:"Application Directory.vi"() -> ("Application Directory"=w381:path)
            n237 = Path To String(path=w381) -> (string=w380:string)
            n238 = Concatenate Strings(w380, "\\Image") -> (w378:string)
            n239 = String To Path(string=w378) -> (path=w376:path)
            n240 = call <vilib>:"Check if File or Folder Exists.vi"("path"=w376) -> ("file or folder exists?"=w377:bool)  [unwired: 8 in, 2 out]
            n241 = case shown="False" w377 {
              tunnel: w376 -> [w383 w384]
              tunnel: [w382 w384] -> w375
              frame False {
                n242 = Create Folder(path (use dialog)=w383) -> (created path=w382:path)  [unwired: 2 in, 2 out]
              }
              frame True {
              }
            }
            n243 = local write "Image Path"(w375) -> ()
          }
        }
      }
      event "Exit": Value Change {
        n244 = event-data() -> ()  [unwired: 1 in, 6 out]
        n245 = flat-sequence {
          tunnel: w385 -> [w388]
          tunnel: w386 -> [w409]
          frame #0 {
            n246 = local read "Acquisition Status"() -> (w391:bool)
            n247 = local read "DeviceHandle"() -> (w390:u64)
            n248 = case shown="True" w391 {
              tunnel: w390 -> [w395 w402]
              tunnel: [w395 w400] -> w389
              tunnel: w388 -> [_ w399]
              frame False {
              }
              frame True {
                n249 = call <vilib>:"Acquire Semaphore.vi"("semaphore"=w399) -> ("semaphore out"=w398:T2)  [unwired: 4 in, 2 out]
                n250 = flat-sequence {
                  tunnel: w402 -> [w403]
                  tunnel: [w403] -> w401
                  tunnel: w398 -> [w404]
                  tunnel: [w404] -> w397
                  tunnel: [w405] -> w400
                  tunnel: w401 -> [w405]
                  tunnel: [w406] -> w396
                  tunnel: w397 -> [w406]
                  frame #0 {
                    n251 = call "StopGrab.vi"("InputHandle"=w403) -> ()  [unwired: 1 in, 3 out]
                  }
                  frame #1 {
                    n252 = local write "Acquisition Status"(FALSE) -> ()
                  }
                }
                n253 = call <vilib>:"Release Semaphore.vi"("semaphore"=w396) -> ()  [unwired: 5 in, 2 out]
              }
            }
            n254 = local read "Open Status"() -> (w392:bool)
            n255 = case shown="True" w392 {
              tunnel: w389 -> [_ w393]
              frame False {
              }
              frame True {
                n256 = call "CloseDevice.vi"("nInputHandle"=w393) -> ()  [unwired: 1 in, 2 out]
                n257 = local write "Open Status"(FALSE) -> ()
              }
            }
          }
          frame #1 {
            n258 = local write "IsExit"(TRUE) -> ()
            n259 = Generate User Event(user event=w409, event data cluster="Quit") -> ()  [unwired: 2 in, 2 out]
          }
        }
      }
      event Panel Close? {
        n260 = event-data() -> ()  [unwired: 1 in, 4 out]
        n261 = flat-sequence {
          tunnel: w411 -> [w414]
          tunnel: w412 -> [w434]
          frame #0 {
            n262 = local read "Acquisition Status"() -> (w417:bool)
            n263 = local read "DeviceHandle"() -> (w416:u64)
            n264 = case shown="True" w417 {
              tunnel: w416 -> [w421 w428]
              tunnel: [w421 w426] -> w415
              tunnel: w414 -> [_ w425]
              frame False {
              }
              frame True {
                n265 = call <vilib>:"Acquire Semaphore.vi"("semaphore"=w425) -> ("semaphore out"=w424:T2)  [unwired: 4 in, 2 out]
                n266 = flat-sequence {
                  tunnel: w428 -> [w429]
                  tunnel: [w429] -> w427
                  tunnel: w424 -> [w430]
                  tunnel: [w430] -> w423
                  tunnel: [w433] -> w426
                  tunnel: w427 -> [w433]
                  tunnel: [w431] -> w422
                  tunnel: w423 -> [w431]
                  frame #0 {
                    n267 = call "StopGrab.vi"("InputHandle"=w429) -> ()  [unwired: 1 in, 3 out]
                  }
                  frame #1 {
                    n268 = local write "Acquisition Status"(FALSE) -> ()
                  }
                }
                n269 = call <vilib>:"Release Semaphore.vi"("semaphore"=w422) -> ()  [unwired: 5 in, 2 out]
              }
            }
            n270 = local read "Open Status"() -> (w418:bool)
            n271 = case shown="True" w418 {
              tunnel: w415 -> [_ w419]
              frame False {
              }
              frame True {
                n272 = call "CloseDevice.vi"("nInputHandle"=w419) -> ()  [unwired: 1 in, 2 out]
                n273 = local write "Open Status"(FALSE) -> ()
              }
            }
          }
          frame #1 {
            n274 = local write "IsExit"(TRUE) -> ()
            n275 = Generate User Event(user event=w434, event data cluster="Quit") -> ()  [unwired: 2 in, 2 out]
          }
        }
        n276 = event-data() -> ()  [unwired: 2 in, 1 out]
      }
    }
    "error out" <- w264
    n277 = call <vilib>:"Simple Error Handler.vi"("error in (no error)"=w264) -> ()  [unwired: 4 in, 5 out]
  }
  n278 = while {
    tunnel: w2 -> [w437]
    stop <- w439 stop-if-true
    # "Configure Refresh Loop"
    n279 = event shown="[3] \"BalanceWhiteAuto\": Value Change" {
      selector: _ -> [_ _ _ _ _]
      dyn-events: _ -> [_ _ _ _ _]
      timeout: _ -> [_ _ _ _ _]
      tunnel: [errorcluster {FALSE, 0, ""} w444 w459 w475 errorcluster {"status"=FALSE, "code"=0, "source"=""} ("错误常量")] -> w438
      tunnel: [FALSE FALSE FALSE FALSE TRUE] -> w439
      tunnel: w437 -> [_ w442 w457 w473 _]
      event Timeout {
        n280 = event-data() -> ()  [unwired: 1 in, 3 out]
      }
      event "ExposureTime": Value Change {
        n281 = event-data() -> ()  [unwired: 1 in, 6 out]
        n282 = local read "DeviceHandle"() -> (w445:u64)
        n283 = Not A Number/Path/Refnum?(number/path/refnum=w445) -> (NaN/Path/Refnum?=w446:bool)
        n284 = case shown="False" w446 {
          tunnel: w445 -> [w449 _]
          tunnel: [w448 errorcluster {TRUE, 5000, "GxSingleCam"}] -> w444
          tunnel: w442 -> [w447 _]
          frame False {
            n285 = flat-sequence {
              tunnel: w449 -> [w452]
              tunnel: [w453] -> w448
              tunnel: w447 -> [w454]
              frame #0 {
                n286 = local read "ExposureTime"() -> (w450:dbl)
                n287 = call "SetFloatValue.vi"("fValue"=w450, "strName"="ExposureTime", "nInputHandle"=w452) -> ("error out"=w453:errorcluster)  [unwired: 1 in, 2 out]
              }
              frame #1 {
                n288 = Generate User Event(user event=w454, event data cluster="UpdateParam") -> ()  [unwired: 2 in, 2 out]
              }
            }
          }
          frame True {
          }
        }
      }
      event "Gain": Value Change {
        n289 = event-data() -> ()  [unwired: 1 in, 6 out]
        n290 = local read "DeviceHandle"() -> (w461:u64)
        n291 = Not A Number/Path/Refnum?(number/path/refnum=w461) -> (NaN/Path/Refnum?=w460:bool)
        n292 = case shown="False" w460 {
          tunnel: w461 -> [w464 _]
          tunnel: [w463 errorcluster {TRUE, 0, "设备句柄无效"}] -> w459
          tunnel: w457 -> [w462 _]
          frame False {
            n293 = flat-sequence {
              tunnel: w464 -> [w467]
              tunnel: [w468] -> w463
              tunnel: w462 -> [w470]
              frame #0 {
                n294 = local read "Gain"() -> (w465:dbl)
                n295 = call "SetFloatValue.vi"("fValue"=w465, "strName"="Gain", "nInputHandle"=w467) -> ("error out"=w468:errorcluster)  [unwired: 1 in, 2 out]
              }
              frame #1 {
                n296 = Generate User Event(user event=w470, event data cluster="UpdateParam") -> ()  [unwired: 2 in, 2 out]
              }
            }
          }
          frame True {
          }
        }
      }
      event "BalanceWhiteAuto": Value Change {
        n297 = event-data() -> ()  [unwired: 1 in, 6 out]
        n298 = local read "DeviceHandle"() -> (w472:u64)
        n299 = Not A Number/Path/Refnum?(number/path/refnum=w472) -> (NaN/Path/Refnum?=w476:bool)
        n300 = case shown="False" w476 {
          tunnel: w472 -> [w479 _]
          tunnel: [w478 errorcluster {TRUE, 0, "设备句柄无效"}] -> w475
          tunnel: w473 -> [w477 _]
          frame False {
            n301 = flat-sequence {
              tunnel: w479 -> [w482]
              tunnel: [w483] -> w478
              tunnel: w477 -> [w484]
              frame #0 {
                n302 = local read "BalanceWhiteAuto"() -> (w480:string)
                n303 = call "SetEnumValueByString.vi"("strValue"=w480, "strName"="BalanceWhiteAuto", "nInputHandle"=w482) -> ("error out"=w483:errorcluster)  [unwired: 1 in, 2 out]
              }
              frame #1 {
                n304 = Generate User Event(user event=w484, event data cluster="UpdateParam") -> ()  [unwired: 2 in, 2 out]
              }
            }
          }
          frame True {
          }
        }
      }
      event "Exit": Value Change {
        n305 = event-data() -> ()  [unwired: 1 in, 6 out]
      }
    }
    n306 = local write "error out"(w438) -> ()
    n307 = call <vilib>:"Simple Error Handler.vi"("error in (no error)"=w438) -> ()  [unwired: 4 in, 5 out]
  }
  n308 = flat-sequence {
    tunnel: w2 -> [w500]
    frame #0 {
      w491 = 0.0
      w492 = ""
      # "Init Param"
      n309 = local write "Acquisition Status"(FALSE) -> ()
      n310 = local write "ImageSaving"(FALSE) -> ()
      n311 = local write "Open Status"(FALSE) -> ()
      n312 = local write "IsExit"(FALSE) -> ()
      n313 = local write "TriggerSource"(w492) -> ()
      n314 = local write "BalanceWhiteAuto"(w492) -> ()
      n315 = local write "ExposureTime"(w491) -> ()
      n316 = local write "TriggerMode"(w492) -> ()
      n317 = local write "Gain"(w491) -> ()
    }
    frame #1 {
      n318 = call "InitLib.vi"() -> ("GX_STATUS"=w495:i32, "error out"=w496:errorcluster)  [unwired: 1 in]
      n319 = case shown="Error" w496 {
        selector: w496 -> [_ w498]
        tunnel: w495 -> [_ w497]
        frame No Error {
        }
        frame Error {
          n320 = call <vilib>:"Simple Error Handler.vi"("error code (no error:0)"=w497, "error in (no error)"=w498) -> ("error?"=w499:bool)  [unwired: 3 in, 4 out]
          n321 = Stop(stop? (T)=w499) -> ()
        }
      }
    }
    frame #2 {
      n322 = Generate User Event(user event=w500, event data cluster="UpdateUI") -> ()  [unwired: 2 in, 2 out]
    }
  }
  n323 = while {
    stop <- w502 stop-if-true
    n324 = local read "DeviceHandle"() -> (w504:u64)
    n325 = Wait (ms)(milliseconds to wait=2000) -> ()  [unwired: 1 out]
    n326 = Not A Number/Path/Refnum?(number/path/refnum=w504) -> (NaN/Path/Refnum?=w503:bool)
    n327 = case shown="False" w503 {
      tunnel: w504 -> [w509 _]
      frame False {
        n328 = local read "BalanceWhiteAuto"() -> (w507:string)
        n329 = Equal?(x=w507, y="Once") -> (x = y?=w506:bool)
        n330 = case shown="True" w506 {
          tunnel: w509 -> [_ w510]
          frame False {
          }
          frame True {
            n331 = local read "IsColor"() -> (w511:bool)
            n332 = case shown="True" w511 {
              tunnel: w510 -> [_ w513]
              frame False {
              }
              frame True {
                n333 = call "GetEnumValue.vi"("nInputHandle"=w513, "strName"="BalanceWhiteAuto") -> ("strCurName"=w512:string)  [unwired: 9 in, 4 out]
                n334 = local write "BalanceWhiteAuto"(w512) -> ()
              }
            }
          }
        }
      }
      frame True {
      }
    }
    n335 = local read "IsExit"() -> (w502:bool)
  }
  n336 = Stop(stop? (T)=w3) -> ()
